vi "getWavelengthDisp.vi"() -> ()   [LabVIEW 2016]
uses:
  <vilib>/Analysis/baseanly.llb/Mean (DBL).vi
  <vilib>/Analysis/NI_AALBase.lvlib
  x32/CLDevIFace.dll
panel:
  in  "Alarm Threshold":dbl=0.0005 format="%#_13g"
  out "Operating 2":bool
  in  "Operate":bool
  out "Locked?":bool
  in  "Set lock point":bool
  out "Wavelength":dbl format="%0.5f"
  out "0.75ppm in Wave (nm)":dbl format="%#_3g"
  out "0.75ppm in Freq (MHz)":dbl
  out "Freq (Hz)":dbl
  out "standard dev":dbl format="%0.5f"
  in  "# for Stdev":i32=7
  in  "Avg":i32=1
  out "Delta MHz":dbl
  in  "Scale Factor":dbl=800.0
  out "Power (mW)":dbl format="%.9f"
  in  "Clear Chart?":bool
  in  "Delay Time (s)":dbl=0.01
  out "Wavelength vs time":cluster{dbl[], dbl[]}(graph)
  out "error out":errorcluster
  out "output param":i32
  in  "stop":bool
  in  "OK Button":bool
  in  "CommPort":dbl=5.0 caption="Comm Port #"
  # "Pr = 605.977 nm"
  # "At start-up:\n1. Lock laser;\n2. Click \"Set lock point\";\n3. Click \"Operate\";\n3. Clear chart.\n\nAt shutdown:\n1. Click operate;\n2. Turn off laser."
  # "Super cavity FSR  6 GHz\nZerodure FSR  750 MHz"
  # "1 pm = 200 MHz @1212nm\n1 pm = 800 MHz @606 nm"
  # "Bristol 621B accuracy = 0.75 ppm\nuseful conversions:"
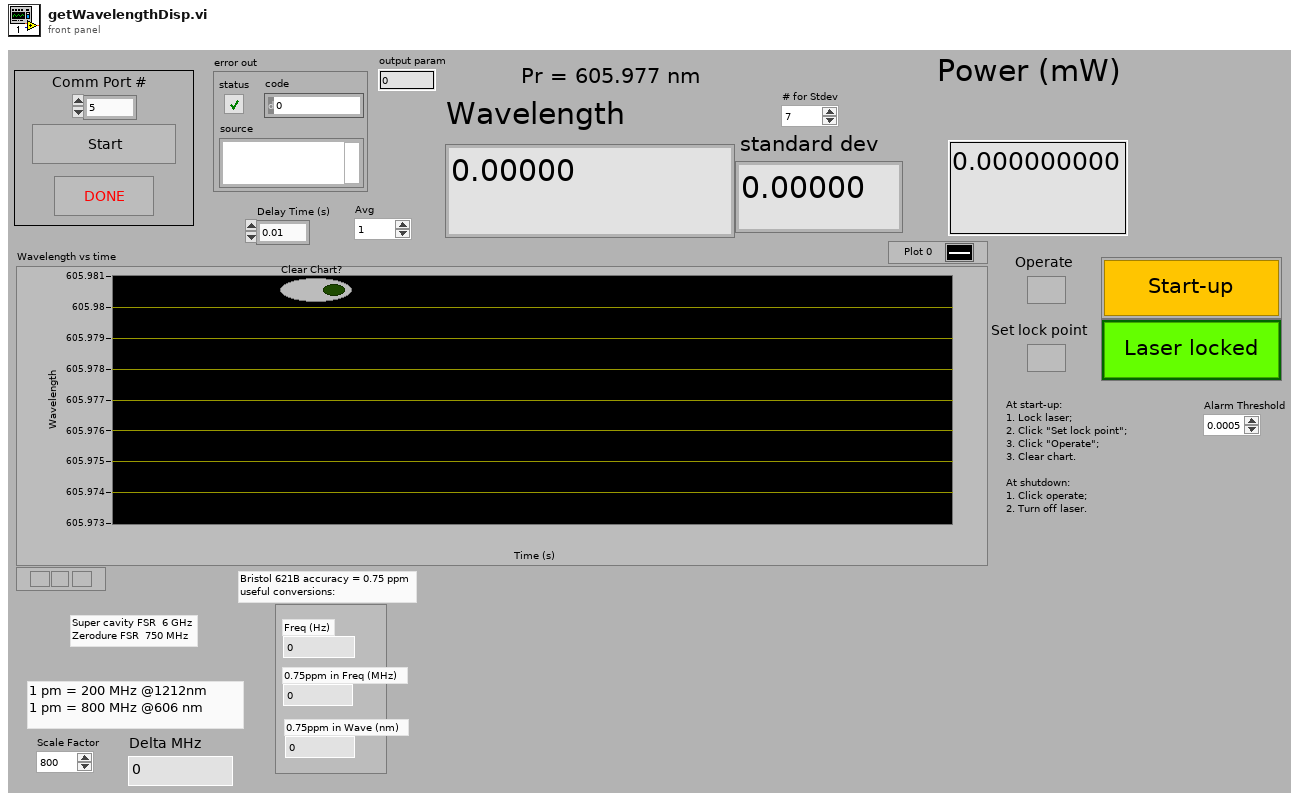
[diagram p1: front panel]
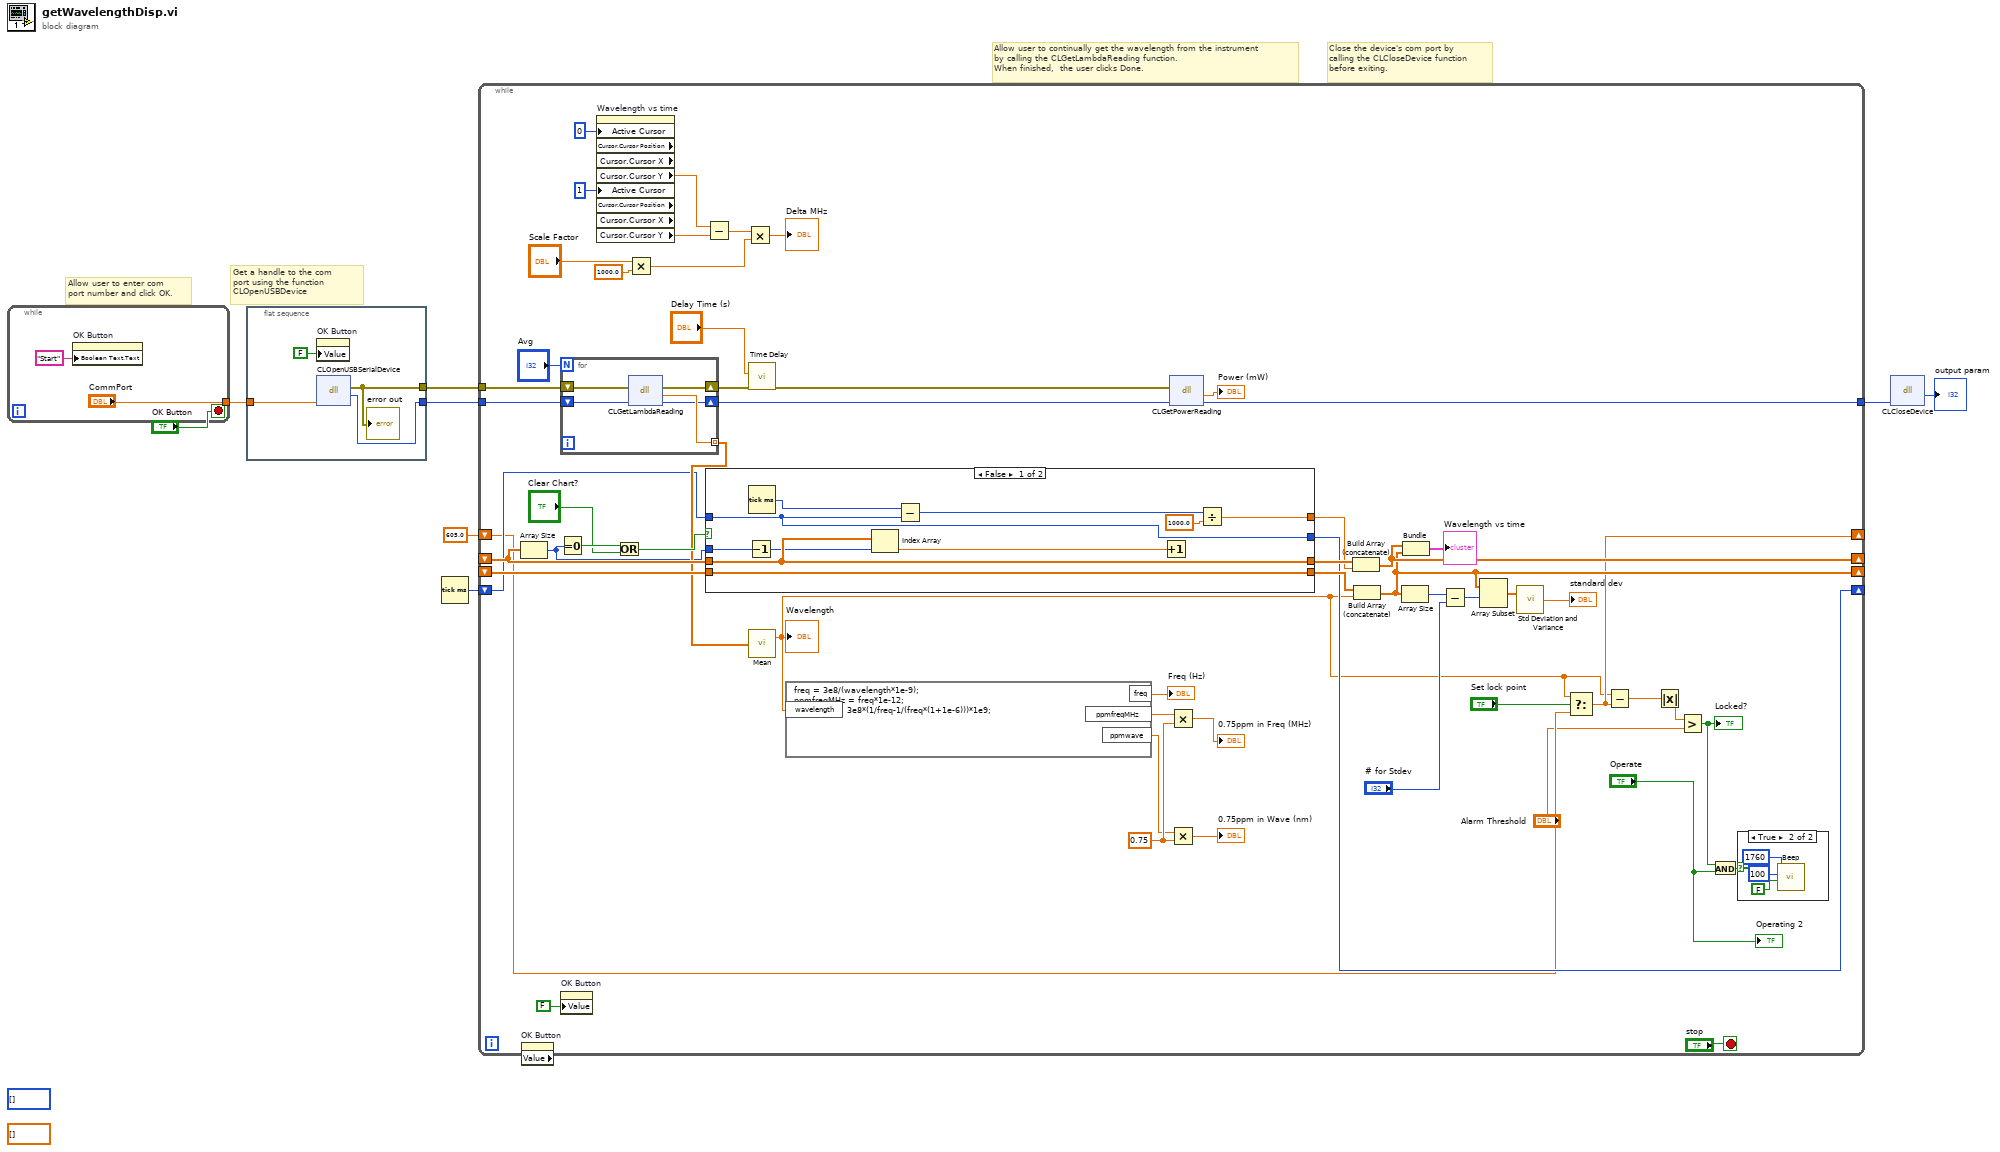
[diagram p0: block diagram]
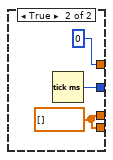
[diagram p3: hidden frame]
diagram:
  (unwired) i32[] []
  (unwired) dbl[] []
  # "Close the device's com port by\ncalling the CLCloseDevice function\nbefore exiting."
  # "Allow user to continually get the wavelength from the instrument\nby calling the CLGetLambdaReading function.  \nWhen finished,  the user clicks Done."
  # "Get a handle to the com\nport using the function CLOpenUSBDevice"
  # "Allow user to enter com \nport number and click OK."
  n1 = while {
    tunnel: ["CommPort"] -> w7
    stop <- "OK Button" stop-if-true
    n2 = property on="OK Button" class="Bool (strict)"("Boolean Text.Text"="Start") -> ()  [unwired: 2 in, 2 out]
  }
  n3 = flat-sequence {
    tunnel: w7 -> [w14]
    tunnel: [w13] -> w6
    tunnel: [w11] -> w3
    frame #0 {
      n4 = property on="OK Button" class="Bool (strict)"("Value"=FALSE) -> ()  [unwired: 2 in, 2 out]
      n5 = dll-call lib="C:/Users/Lab/Desktop/AFCgit/AFC-code/HardWare/LabView/Wavemeter/x32/CLDevIFace.dll" fn="CLOpenUSBSerialDevice"("commPort"=w14) -> (error out=w11:errorcluster, "return type"=w13:i32)  [unwired: 4 in, 1 out]
      "error out" <- w11
    }
  }
  n6 = Tick Count (ms)() -> (millisecond timer value=w2:u32)
  n7 = while {
    tunnel: w6 -> [w70]
    tunnel: [w58] -> w5
    shift-right: [w38] -> _
    shift-left: _ -> [w62]
    shift-right: [w67] -> _
    shift-left: _ -> [w43]
    tunnel: w3 -> [w63]
    shift-right: [w26] -> _
    shift-left: w2 -> [w27]
    shift-right: [w24] -> _
    shift-left: 605.0 ("mean") -> [w23]
    stop <- "stop" stop-if-true
    w30 = 0.75 ("y")
    n8 = Array Size(array=w43) -> (size(s)=w40:i32)
    n9 = property on="OK Button" class="Bool (strict)" props=["Value"]() -> ()  [unwired: 2 in, 3 out]
    n10 = Equal To 0?(x=w40) -> (x = 0?=w48:bool)
    n11 = for {
      N: "Avg" -> [_]
      tunnel: [w77] -> w41 mode=indexing
      shift-right: [w74] -> w59
      shift-left: w70 -> [w78]
      shift-right: [w76] -> w64
      shift-left: w63 -> [w75]
      n12 = dll-call lib="C:/Users/Lab/Desktop/AFCgit/AFC-code/HardWare/LabView/Wavemeter/x32/CLDevIFace.dll" fn="CLGetLambdaReading"(error in=w75, "devHandle"=w78) -> (error out=w76:errorcluster, "return type"=w77:dbl, "devHandle"=w74:i32)  [unwired: 2 in, 1 out]
    }
    n13 = property on="OK Button" class="Bool (strict)"("Value"=FALSE) -> ()  [unwired: 2 in, 2 out]
    n14 = property on="Wavelength vs time" class="XYGraph (strict)" props=["Active Cursor", "Cursor", "Cursor Position", "Cursor", "Cursor X", "Cursor", "Cursor Y", "Active Cursor", "Cursor", "Cursor Position", "Cursor", "Cursor X", "Cursor", "Cursor Y"]("Active Cursor"=u32 0, "Active Cursor"=u32 1) -> ("Cursor.Cursor Y"=w54:dbl, "Cursor.Cursor Y"=w55:dbl)  [unwired: 2 in, 6 out]
    n15 = Or(x=w48, y="Clear Chart?") -> (x .or. y?=w46:bool)
    n16 = Multiply(x="Scale Factor", y=1000.0) -> (x*y=w49:dbl)
    n17 = Subtract(x=w54, y=w55) -> (x-y=w56:dbl)
    n18 = case shown="False" w46 {
      tunnel: w62 -> [w88 _]
      tunnel: w43 -> [w87 _]
      tunnel: [w87 w89] -> w44
      tunnel: [w88 w89] -> w45
      tunnel: w40 -> [w85 _]
      tunnel: [w80 0] -> w39
      tunnel: w27 -> [w79 _]
      tunnel: [w79 w90] -> w26
      frame False {
        n19 = Decrement(x=w85) -> (x-1=w84:i32)
        n20 = Tick Count (ms)() -> (millisecond timer value=w83:u32)
        n21 = Index Array(array=w87, index=w84) -> (element=w86:dbl)
        n22 = Subtract(x=w83, y=w79) -> (x-y=w81:u32)
        n23 = Increment(x=w86) -> ()  [unwired: 1 out]
        n24 = Divide(x=w81, y=1000.0) -> (x/y=w80:dbl)
      }
      frame True {
        w89 = dbl[] []
        n25 = Tick Count (ms)() -> (millisecond timer value=w90:u32)
      }
    }
    n26 = Multiply(x=w56, y=w49) -> (x*y=→"Delta MHz":dbl)
    n27 = call "Time Delay"("error in (no error)"=w64, "Delay Time (s)"="Delay Time (s)") -> ("error out"=w61:errorcluster)  [unwired: 9 in]
    n28 = call-poly <vilib>:"Mean.vi"("X"=w41) -> ("mean"=w18:dbl)  [unwired: 1 out]
    "Wavelength" <- w18
    n29 = formula code="freq = 3e8/(wavelength*1e-9);\nppmfreqMHz = freq*1e-12;\nppmwave = 3e8*(1/freq-1/(freq*(1+1e-6)))*1e9;"("wavelength"=w18) -> ("freq"=→"Freq (Hz)":dbl, "ppmfreqMHz"=w32:dbl, "ppmwave"=w29:dbl)
    n30 = dll-call lib="C:/Users/Lab/Desktop/AFCgit/AFC-code/HardWare/LabView/Wavemeter/x32/CLDevIFace.dll" fn="CLGetPowerReading"(error in=w61, "devHandle"=w59) -> ("return type"=→"Power (mW)":dbl, "devHandle"=w58:i32)  [unwired: 2 in, 2 out]
    n31 = Multiply(x=w32, y=w30) -> (x*y=→"0.75ppm in Freq (MHz)":dbl)
    n32 = Multiply(x=w29, y=w30) -> (x*y=→"0.75ppm in Wave (nm)":dbl)
    n33 = Build Array (concatenate)(w44, w39) -> (w67:dbl[])
    n34 = Build Array (concatenate)(w45, w18) -> (w38:dbl[])
    n35 = Array Size(array=w38) -> (size(s)=w37:i32)
    n36 = Bundle(w67, w38) -> (→"Wavelength vs time":cluster{dbl[], dbl[]})  [unwired: 1 in]
    n37 = Subtract(x=w37, y="# for Stdev") -> (x-y=w35:i32)
    n38 = Array Subset(array=w38, index=w35) -> (w34:dbl[])  [unwired: 1 in]
    n39 = call <vilib>:"Std Deviation and Variance.vi"("X"=w34) -> ("standard deviation"=→"standard dev":dbl)  [unwired: 1 in, 2 out]
    n40 = Select(t=w18, s="Set lock point", f=w23) -> (s? t:f=w24:dbl)
    n41 = Subtract(x=w18, y=w24) -> (x-y=w20:dbl)
    n42 = Absolute Value(x=w20) -> (abs(x)=w19:dbl)
    n43 = Greater?(x=w19, y="Alarm Threshold") -> (0:w15:bool)
    "Locked?" <- w15
    n44 = And(x=w15, y="Operate") -> (x .and. y?=w17:bool)
    n45 = case shown="True" w17 {
      frame False {
      }
      frame True {
        n46 = call <vilib>:"Beep.vi"("use system alert? (T)"=FALSE, "duration (msec)"=u32 100, "frequency (Hz)"=u32 1760) -> ()  [unwired: 9 in]
      }
    }
    "Operating 2" <- "Operate"
  }
  n47 = dll-call lib="C:/Users/Lab/Desktop/AFCgit/AFC-code/HardWare/LabView/Wavemeter/x32/CLDevIFace.dll" fn="CLCloseDevice"("commPort"=w5) -> ("return type"=→"output param":i32)  [unwired: 4 in, 2 out]
